vi "Receive Value Change Event.vi"(8 "error in (no error)":errorcluster, 10 "ValueChangeMsg":refnum<class "ValueChangeMsg.lvclass">, 11 "OneButtonDialogBox in":refnum<class "OneButtonDialogBox.lvclass">) -> (0 "error out":errorcluster, 3 "OneButtonDialogBox out":refnum<class "OneButtonDialogBox.lvclass">)   [LabVIEW 2020, in "MVA Framework.lvlib" / "OneButtonDialogBox.lvlib" / "OneButtonDialogBox.lvclass"]
doc: "接收值改变事件"
uses:
  OneButtonDialogBox.lvclass
  C:/Program Files/National Instruments/LabVIEW 2020/vi.lib/ActorFramework/Actor/Actor.lvclass
  modules/mva-viewable/Source/ActorEvents/IEventAggregator Messages/ValueChangeMsg/ValueChangeMsg.lvclass
  <vilib>/ActorFramework/Actor/Actor.lvclass/Actor.ctl
  <vilib>/ActorFramework/Message Enqueuer/Message Enqueuer.lvclass/Message Enqueuer.ctl
  OneButtonDialogBox.lvclass/OneButtonDialogBox.ctl
  <vilib>/ActorFramework/Message Enqueuer/Init from Existing Queue.vi
  <vilib>/ActorFramework/Message Enqueuer/Enqueue.vi
  <vilib>/ActorFramework/Stop Msg/Stop Msg.lvclass
  C:/Program Files/National Instruments/LabVIEW 2020/vi.lib/ActorFramework/Message/Message.lvclass
  <vilib>/ActorFramework/Message Priority Queue/Priority Enqueue.vi
  <vilib>/ActorFramework/Message Enqueuer/Message Enqueuer.lvclass
  IDialogBox/IDialogBox Messages/Dialog Return Msg/Dialog Return Msg.lvclass
  <vilib>/ActorFramework/Actor/Actor.lvclass
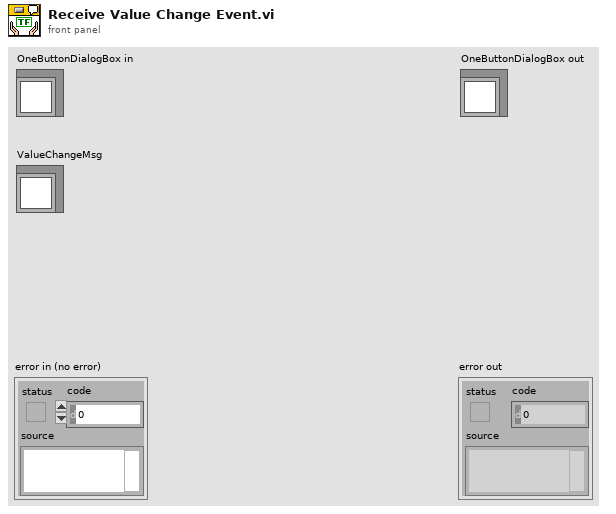
[diagram p1: front panel]
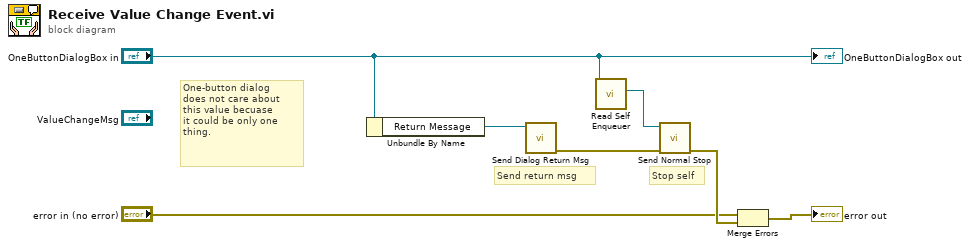
[diagram p0: block diagram]
diagram:
  # "One-button dialog\ndoes not care about\nthis value becuase\nit could be only one\nthing."
  # "Stop self"
  # "Send return msg"
  n1 = Unbundle By Name("OneButtonDialogBox in") -> ("Return Message"=w1:refnum<class "Dialog Return Msg.lvclass">)
  n2 = call "Send Dialog Return Msg.vi"("Dialog Return Msg"=w1) -> ("error out"=w6:errorcluster)  [unwired: 10 in]
  n3 = call <vilib>:"Read Self Enqueuer.vi"("Actor"="OneButtonDialogBox in") -> ("Self Enqueuer"=w7:refnum<class "Message Enqueuer.lvclass">)  [unwired: 10 in]
  n4 = call <vilib>:"Send Normal Stop.vi"("error in (no error)"=w6, "Message Enqueuer"=w7) -> ("error out"=w4:errorcluster)  [unwired: 9 in]
  n5 = Merge Errors("error in (no error)", w4) -> (→"error out":errorcluster)
  "OneButtonDialogBox out" <- "OneButtonDialogBox in"
